vi "Climb_Test.vi"(11 "Joystick_In":T1) -> ()   [LabVIEW 2019]
uses:
  Utility_VIs/Joystick_Controls.ctl
  Subsystems/Climb/Climb_Cluster.ctl
  Globals/Climb_Globals.vi
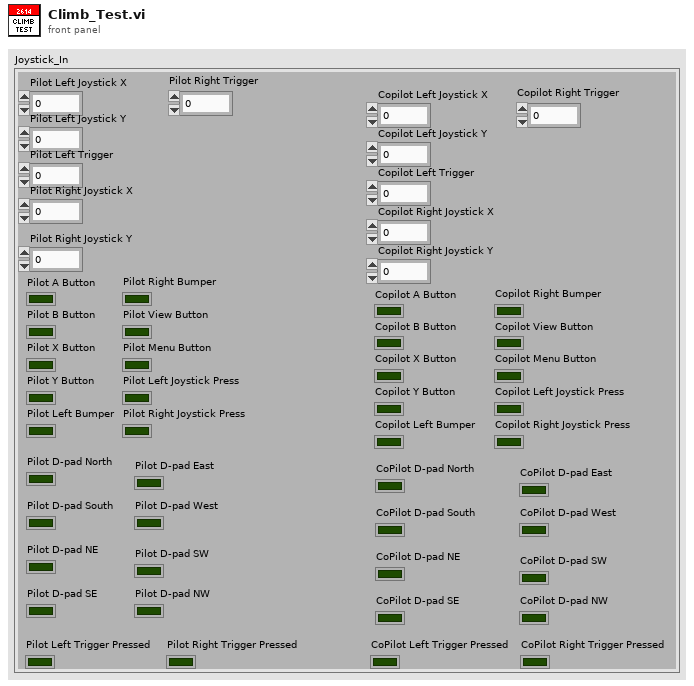
[diagram p1: front panel]
types:
  T1 = typedef "Joystick_Controls.ctl" = cluster{"Pilot Left Joystick X":dbl, "Pilot Left Joystick Y":dbl, "Pilot A Button":bool, "Pilot B Button":bool, "Pilot X Button":bool, "Pilot Y Button":bool, "Pilot Left Bumper":bool, "Pilot Right Bumper":bool, "Pilot View Button":bool, "Pilot Menu Button":bool, "Pilot Left Joystick Press":bool, "Pilot Right Joystick Press":bool, "Pilot Left Trigger":dbl, "Pilot Right Joystick X":dbl, "Pilot Right Joystick Y":dbl, "Pilot Right Trigger":dbl, "Copilot Left Joystick X":dbl, "Copilot Left Joystick Y":dbl, "Copilot A Button":bool, "Copilot B Button":bool, "Copilot X Button":bool, "Copilot Y Button":bool, "Copilot Left Bumper":bool, "Copilot Right Bumper":bool, "Copilot View Button":bool, "Copilot Menu Button":bool, "Copilot Left Joystick Press":bool, "Copilot Right Joystick Press":bool, "Copilot Left Trigger":dbl, "Copilot Right Joystick X":dbl, "Copilot Right Joystick Y":dbl, "Copilot Right Trigger":dbl, "Pilot D-pad North":bool, "Pilot D-pad South":bool, "Pilot D-pad East":bool, "Pilot D-pad West":bool, "Pilot D-pad NE ":bool, "Pilot D-pad SE":bool, "Pilot D-pad SW":bool, "Pilot D-pad NW":bool, "CoPilot D-pad North":bool, "CoPilot D-pad South":bool, "CoPilot D-pad East":bool, "CoPilot D-pad West":bool, "CoPilot D-pad NE":bool, "CoPilot D-pad SE":bool, "CoPilot D-pad SW":bool, "CoPilot D-pad NW":bool, "Pilot Left Trigger Pressed":bool, "Pilot Right Trigger Pressed":bool, "CoPilot Left Trigger Pressed":bool, "CoPilot Right Trigger Pressed":bool}
  T2 = typedef "Climb_Cluster.ctl" = cluster{"Control_State":enum16{"No-Op", "Extending", "Clamping", "Balancing", "Manual_Control"}, "Extend_Climber?":bool, "Clamp?":bool, "Balance?":bool, "Transverse_Throttle":dbl, "Elevator_Throttle":dbl, "Control_Panel_Setpoint?":bool, "Auto-Balance":bool, "Pivot_Throttle":dbl}
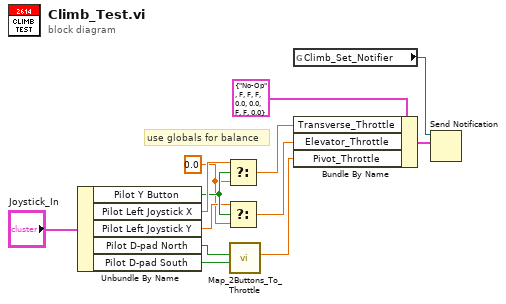
[diagram p0: block diagram]
diagram:
  w6 = 0.0 ("f")
  # "use globals for balance"
  n1 = Unbundle By Name("Joystick_In") -> ("Pilot Y Button"=w8:bool, "Pilot Left Joystick X"=w9:dbl, "Pilot Left Joystick Y"=w7:dbl, "Pilot D-pad North"=w3:bool, "Pilot D-pad South"=w2:bool)
  n2 = Select(t=w9, s=w8, f=w6) -> (s? t:f=w5:dbl)
  n3 = Select(t=w7, s=w8, f=w6) -> (s? t:f=w4:dbl)
  n4 = call "Map_2Buttons_To_Throttle.vi"("Down"=w2, "Up"=w3) -> ("Throttle"=w1:dbl)  [unwired: 9 in]
  n5 = global read "Climb_Globals.vi" "Climb_Set_Notifier"() -> (w12:refnum<notifier>)
  n6 = Bundle By Name(cluster=T2 {"Control_State"=enum."No-Op", "Extend_Climber?"=FALSE, "Clamp?"=FALSE, "Balance?"=FALSE, "Transverse_Throttle"=0.0, "Elevator_Throttle"=0.0, "Control_Panel_Setpoint?"=FALSE, "Auto-Balance"=FALSE, "Pivot_Throttle"=0.0} ("notification"), "Transverse_Throttle"=w5, "Elevator_Throttle"=w4, "Pivot_Throttle"=w1) -> (w10:T2)
  n7 = Send Notification(notification=w10, notifier=w12) -> ()  [unwired: 1 in, 2 out]
